vi "newDataEvent.vi"(8 "error in (no error)":errorcluster, 10 "data":variant, 11 "AnalysisResultsViewer in":refnum<class "AnalysisResultsViewer.lvclass">) -> (0 "error out":errorcluster, 3 "AnalysisResultsViewer out":refnum<class "AnalysisResultsViewer.lvclass">)   [LabVIEW 2009, in "Views.lvlib" / "Camera.lvlib" / "AnalysisResultsViewer.lvclass"]
uses:
  AnalysisResultsViewer.lvclass
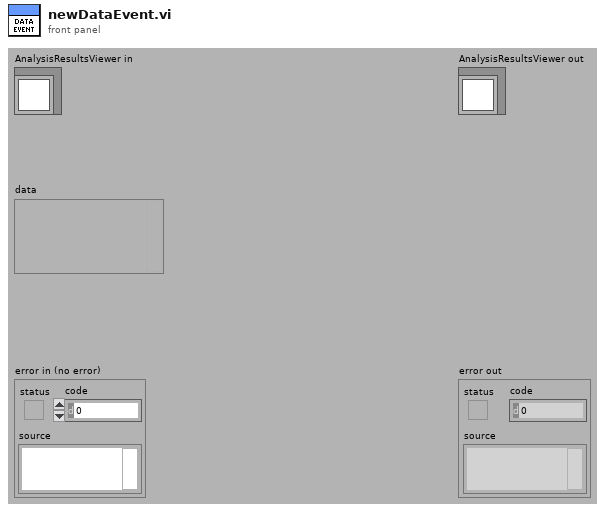
[diagram p1: front panel]
types:
  T1 = cluster{"Name":string, "Results":dbl[], "AnalysisType":string}
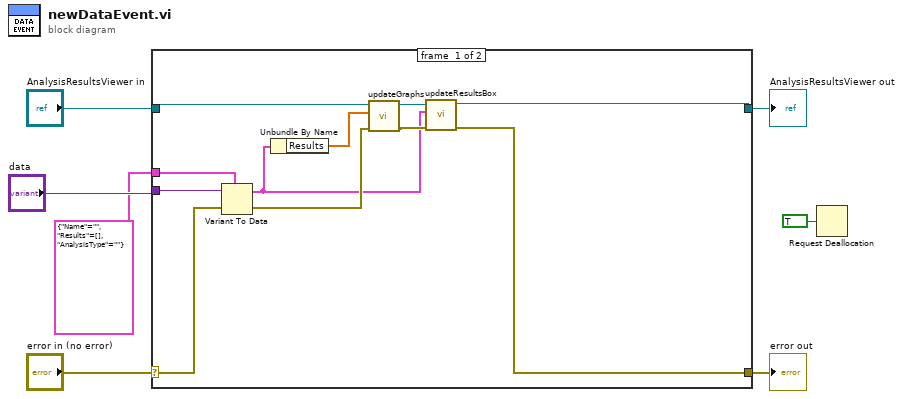
[diagram p0: block diagram]
diagram:
  n1 = case shown="No Error" "error in (no error)" {
    selector: "error in (no error)" -> [w17 w20]
    tunnel: [w9 w20] -> w6
    tunnel: [w10 w19] -> w4
    tunnel: "AnalysisResultsViewer in" -> [w16 w19]
    tunnel: "data" -> [w18 _]
    tunnel: T1 {"Name"="", "Results"=[], "AnalysisType"=""} ("output cluster") -> [w14 _]
    frame #0 {
      n2 = Variant To Data(error in=w17, Variant=w18, type=w14) -> (error out=w15:errorcluster, data=w8:T1)
      n3 = Unbundle By Name(w8) -> ("Results"=w13:dbl[])
      n4 = call "updateGraphs.vi"("error in (no error)"=w15, "Array"=w13, "AnalysisResultsViewer in"=w16) -> ("error out"=w11:errorcluster, "AnalysisResultsViewer out"=w12:refnum<class "AnalysisResultsViewer.lvclass">)  [unwired: 7 in]
      n5 = call "updateResultsBox.vi"("error in (no error)"=w11, "results"=w8, "AnalysisResultsViewer in"=w12) -> ("error out"=w9:errorcluster, "AnalysisResultsViewer out"=w10:refnum<class "AnalysisResultsViewer.lvclass">)  [unwired: 7 in]
    }
    frame #1 {
    }
  }
  "error out" <- w6
  "AnalysisResultsViewer out" <- w4
  n6 = Request Deallocation(TRUE ("flag")) -> ()
